vi "chamber_in.vi"   [LabVIEW 2013]
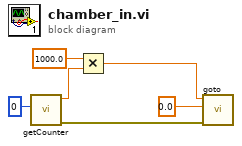
[diagram p0: block diagram]
diagram:
  n1 = call "getCounter.vi"("channel"=0) -> ("错误输出"=w6:errorcluster, "result"=w3:dbl)  [unwired: 9 in]
  n2 = Multiply(x=1000.0, y=w3) -> (x*y=w1:dbl)
  n3 = call "goto.vi"("错误输入（无错误）"=w6, "Y(mm)"=0.0, "X(mm)"=w1) -> ()  [unwired: 8 in, 1 out]
